vi "GetTestsFromPackedProjectLibrary.vi"(0 "Packed Project Library Path":path, 11 "error in (no error)":errorcluster) -> (4 "Tests":path[](array[path]), 6 "Qualified Names":string[](array[string]), 15 "error out":errorcluster)   [LabVIEW 2016, in "Drona.lvlib"]
doc: "Returns the qualified names and test paths of the exported files in packed project library"
uses:
  Drona.lvlib
  <vilib>/Utility/LVLibp/NI_PackedLibraryUtility.lvlib
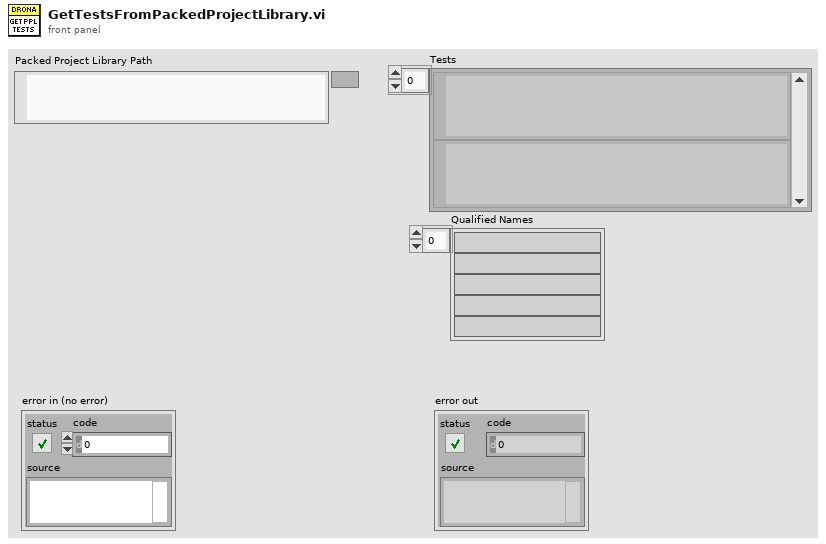
[diagram p1: front panel]
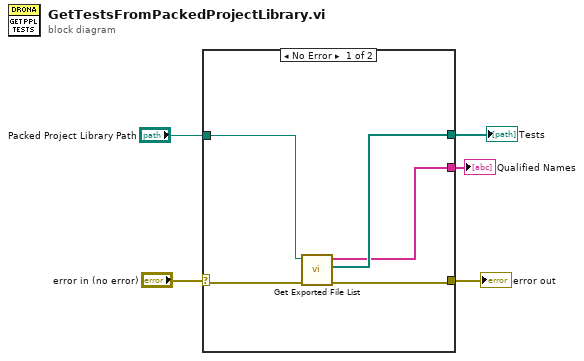
[diagram p0: block diagram]
diagram:
  n1 = case shown="No Error" "error in (no error)" {
    selector: "error in (no error)" -> [w10 w11]
    tunnel: [w7 w11] -> w4
    tunnel: "Packed Project Library Path" -> [w9 _]
    tunnel: [w8 _] -> w2
    tunnel: [w6 _] -> w1
    frame No Error {
      n2 = call <vilib>:"Get Exported File List.vi"("error in (no error)"=w10, "packed library path"=w9) -> ("error out"=w7:errorcluster, "paths"=w8:path[], "qualified names"=w6:string[])  [unwired: 7 in]
    }
    frame Error {
    }
  }
  "error out" <- w4
  "Tests" <- w2
  "Qualified Names" <- w1
